vi "GetPWMmode.vi"(0 "VISA Refnum in":refnum<visa-resource-name>, 2 "Address":u8, 3 "error in (no error)":errorcluster) -> (5 "VISA Refnum out":refnum<visa-resource-name>, 6 "Valid":bool, 7 "mode":u8, 8 "error out":errorcluster)   [LabVIEW 2015, in "Ion Motion Roboclaw.lvlib"]
uses:
  <instrlib>/Ion Motion Roboclaw/Ion Motion Roboclaw.lvlib
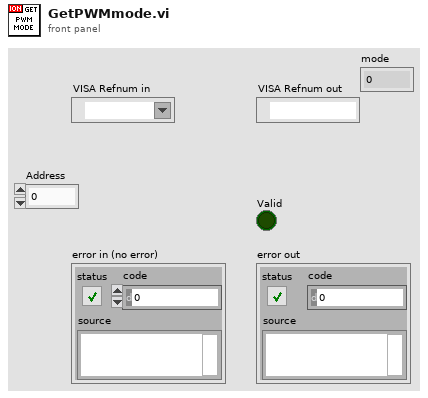
[diagram p1: front panel]
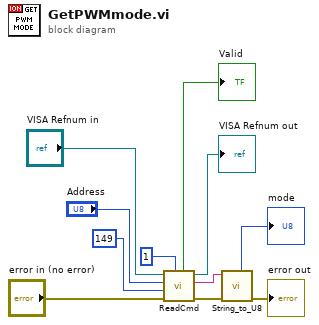
[diagram p0: block diagram]
diagram:
  n1 = call <instrlib>:"ReadCmd.vi"("Read Count"=u32 1, "error in (no error)"="error in (no error)", "Cmd"=u8 149, "Address"="Address", "VISA Refnum in"="VISA Refnum in") -> ("error out"=w9:errorcluster, "Output"=w8:string, "VISA Refnum out"=→"VISA Refnum out":refnum<visa-resource-name>, "Valid"=→"Valid":bool)  [unwired: 3 in]
  n2 = call <instrlib>:"String_to_U8.vi"("error in (no error)"=w9, "String"=w8) -> ("error out"=→"error out":errorcluster, "Argument"=→"mode":u8)  [unwired: 5 in, 1 out]
